vi "Configure Error Handler.vi"(8 "error in (no error)":errorcluster, 11 "Error Handler in":refnum<class "Error Handler.lvclass">) -> (0 "error out":errorcluster, 3 "Error Handler out":refnum<class "Error Handler.lvclass">)   [LabVIEW 2020, in "Error Handler.lvclass"]
uses:
  Error Handler.lvclass
  C:/Git/astemes-lunit/source/Application Framework/Process Classes/Process/Process.lvclass
  Process/Process.lvclass/Process.ctl
  Process/Process.lvclass
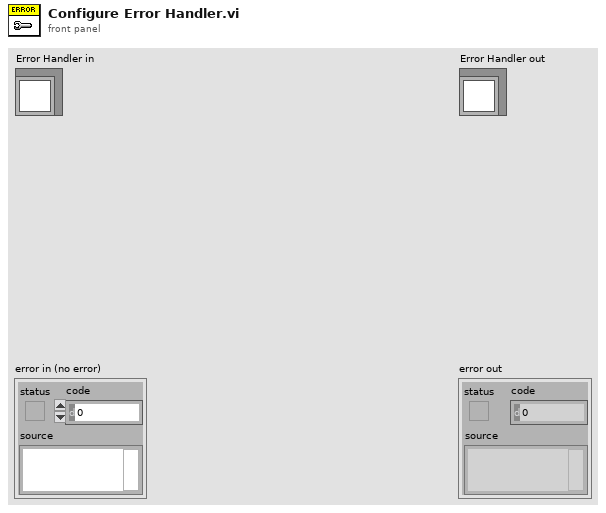
[diagram p1: front panel]
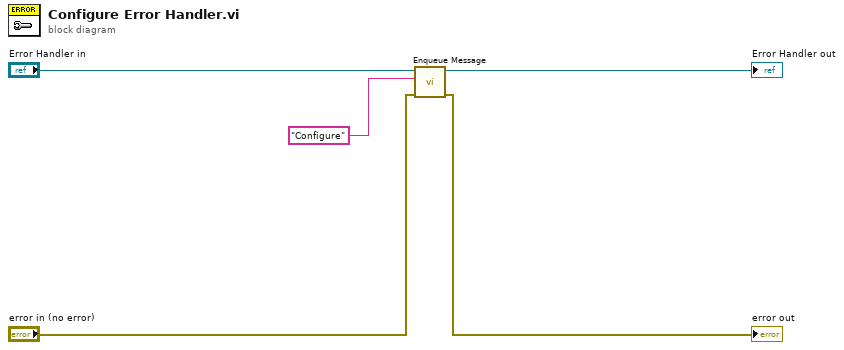
[diagram p0: block diagram]
diagram:
  n1 = call "Enqueue Message.vi"("error in (no error)"="error in (no error)", "Message"="Configure", "Process In"="Error Handler in") -> ("error out"=→"error out":errorcluster, "Process Out"=→"Error Handler out":refnum<class "Error Handler.lvclass">)  [unwired: 7 in]
